vi "S7COMM - Evaluate Response Error Code.vi"(8 "error in (no error)":errorcluster, 11 "Error Code":u16 format="0x%04x") -> (0 "error out":errorcluster)   [LabVIEW 2014, in "S7NetCom.lvclass"]
uses:
  S7NetCom.lvclass
  S7COMM - Response Error Codes--ring.ctl
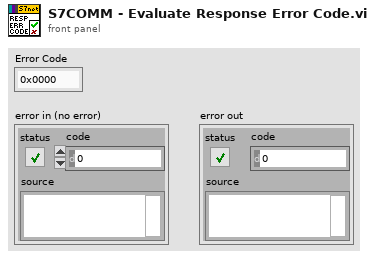
[diagram p1: front panel]
types:
  T1 = typedef "S7NetCom.lvclass/S7COMM - Response Error Codes--ring.ctl" = enum16{"No error (0x0000)"}
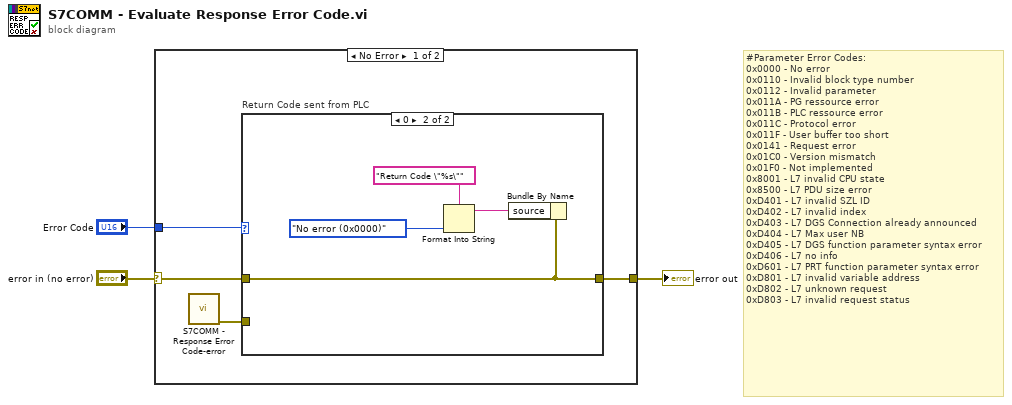
[diagram p0: block diagram]
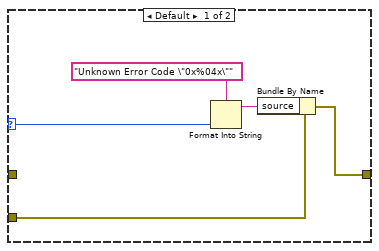
[diagram p2: hidden frame]
diagram:
  # "#Parameter Error Codes:\n0x0000 - No error\n0x0110 - Invalid block type number\n0x0112 - Invalid parameter\n0x011A - PG ressource error\n0x011B - PLC ressource error\n0x011C - Protocol error\n0x011F - User buffer too short\n0x0141 - Request error\n0x01C0 - Version mismatch\n0x01F0 - Not implemented\n0x8001 - L7 invalid CPU state\n0x8500 - L7 PDU size error\n0xD401 - L7 invalid SZL ID\n0xD402 - L7 invalid index\n0xD403 - L7 DGS Connection already announced\n0xD404 - L7 Max user NB\n0xD405 - L7 DGS function parameter syntax error\n0xD406 - L7 no info\n0xD601 - L7 PRT function parameter syntax error\n0xD801 - L7 invalid variable address\n0xD802 - L7 unknown request\n0xD803 - L7 invalid request status"
  n1 = case shown="No Error" "error in (no error)" {
    selector: "error in (no error)" -> [w6 w17]
    tunnel: [w5 w17] -> w3
    tunnel: "Error Code" -> [w7 _]
    frame No Error {
      n2 = call "S7COMM - Response Error Code-error.vi"() -> ("error out"=w4:errorcluster)  [unwired: 11 in]
      n3 = case "Return Code sent from PLC" shown="0" w7 {
        selector: w7 -> [w8 _]
        tunnel: w6 -> [_ w13]
        tunnel: [w11 w13] -> w5
        tunnel: w4 -> [w12 _]
        frame Default {
          n4 = Format Into String(format string="Unknown Error Code \"0x%04x\"", w8) -> (resulting string=w10:string)  [unwired: 2 in, 1 out]
          n5 = Bundle By Name(cluster=w12, "source"=w10) -> (w11:errorcluster)
        }
        frame 0 {
          n6 = Format Into String(format string="Return Code \"%s\"", S7COMM_-_Response_Error_Codes--ring."No error (0x0000)" ("Response Error Codes")) -> (resulting string=w16:string)  [unwired: 2 in, 1 out]
          n7 = Bundle By Name(cluster=w13, "source"=w16) -> ()  [unwired: 1 out]
        }
      }
    }
    frame Error {
    }
  }
  "error out" <- w3
